vi "Init_Instr.vi"(8 "error in (no error)":errorcluster caption="entrée d'erreur (pas d'erreur)", 11 "Class Instrument Firebase Altyor en entrée":refnum<class "Class Instrument Firebase Altyor.lvclass">) -> (0 "error out":errorcluster caption="sortie d'erreur", 3 "Class Instrument Firebase Altyor en sortie":refnum<class "Class Instrument Firebase Altyor.lvclass">)   [LabVIEW 2020, in "Library Instrument & Equipement.lvlib" / "Library Instruments.lvlib" / "Class Instrument Firebase Altyor.lvclass"]
uses:
  Class Instrument Firebase Altyor.lvclass
  Class Instrument Firebase Altyor.lvclass/Class Instrument Firebase Altyor.ctl
  Firebase/Source/Firebase PCBA/Firebase Benches.lvclass
  C:/Users/ngarcin/OneDrive - Altyor/Standard TB/Class/Firebase/Source/Firebase Altyor/Firebase Altyor.lvclass
  Firebase/Source/Firebase AssembledProducts/Firebase AssembledProducts.lvclass
  Firebase/Source/Firebase Benches P2193/Firebase Benches P2193.lvclass
  Firebase/Source/Firebase Altyor/Firebase Altyor.lvclass
  C:/Users/ngarcin/OneDrive - Altyor/Standard TB/Class/Firebase/Source/Firebase Driver/Firebase Driver.lvclass
  Instrument (Default)/Class Instrument (Default).lvclass
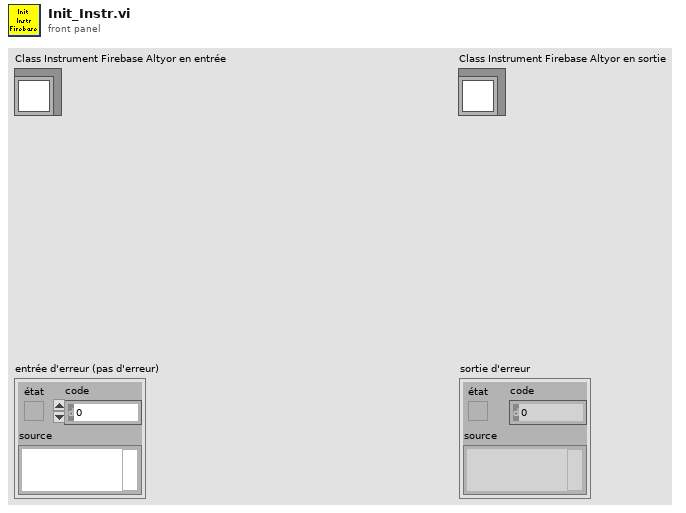
[diagram p1: front panel]
types:
  T1 = typedef "Library Commun.lvlib/Bench Type.ctl" = enum16{"Bench PCBA", "Bench Camera", "Bench Assembly", "Bench PCBA P2193"}
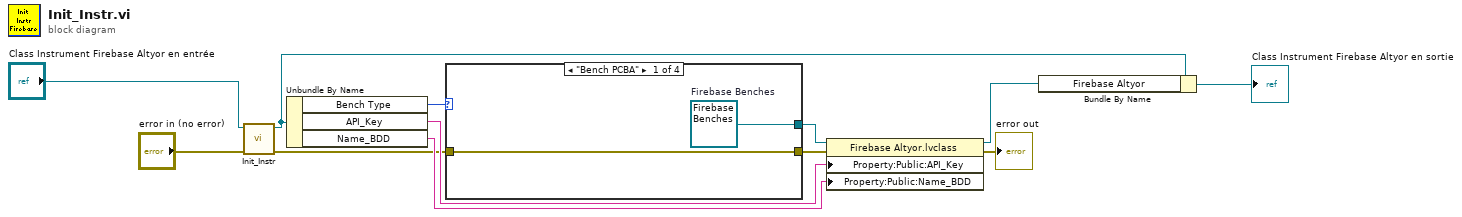
[diagram p0: block diagram]
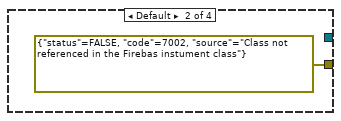
[diagram p2: hidden frame]
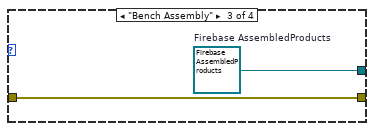
[diagram p3: hidden frame]
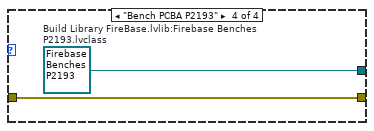
[diagram p4: hidden frame]
diagram:
  n1 = call-parent "Init_Instr.vi"("error in (no error)"="error in (no error)", "Class Instrument (Default) en entrée"="Class Instrument Firebase Altyor en entrée") -> ("error out"=w4:errorcluster, "Class Instrument (Default) en sortie"=w3:refnum<class "Class Instrument Firebase Altyor.lvclass">)  [unwired: 8 in]
  n2 = Unbundle By Name(w3) -> ("Bench Type"=w6:T1, "API_Key"=w10:string, "Name_BDD"=w9:string)
  n3 = case shown="\"Bench PCBA\"" w6 {
    tunnel: [w14 _ w17 w19] -> w7
    tunnel: w4 -> [w13 _ w16 w18]
    tunnel: [w13 errorcluster {"status"=FALSE, "code"=7002, "source"="Class not referenced in the Firebas instument class"} ("error out") w16 w18] -> w5
    frame "Bench PCBA" {
      w14 = refnum<class "Firebase Benches.lvclass"> refnum  # Firebase Benches
    }
    frame Default {
    }
    frame "Bench Assembly" {
      w17 = refnum<class "Firebase AssembledProducts.lvclass"> refnum  # Firebase AssembledProducts
    }
    frame "Bench PCBA P2193" {
      w19 = refnum<class "Firebase Benches P2193.lvclass"> refnum  # Build Library FireBase.lvlib:Firebase Benches P2193.lvclass
    }
  }
  n4 = property class="Firebase Altyor.lvclass"(reference=w7, error in=w5, "Property:Public:API_Key"=w10, "Property:Public:Name_BDD"=w9) -> (reference out=w8:refnum<class "Firebase Altyor.lvclass">, error out=→"error out":errorcluster)
  n5 = Bundle By Name(cluster=w3, "Firebase Altyor"=w8) -> (→"Class Instrument Firebase Altyor en sortie":refnum<class "Class Instrument Firebase Altyor.lvclass">)
